vi "Calibration_Test Target_1mm.vi"   [LabVIEW 2016]
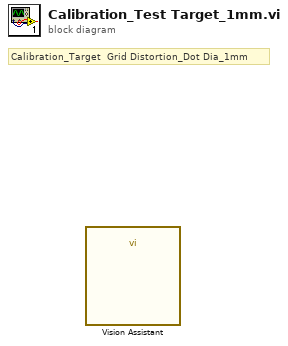
[diagram p0: block diagram]
diagram:
  # "Calibration_Target  Grid Distortion_Dot Dia_1mm"
  n1 = call "Vision Assistant"() -> ()  [unwired: 26 in, 2 out]
